vi "lead-lowPass_v8.vi"(7 "Enable?":bool, 9 "Denominator":fxp<+/-,18,3>[](array[numeric])=[0.0, 0.0], 10 "Numerator":fxp<+/-,18,3>[](array[numeric])=[0.0, 0.0], 11 "Input":fxp<+/-,25,4>) -> (3 "Output":fxp<+/-,25,4> format="%.29g")   [LabVIEW 2017, in "FPGA Controllers.lvlib"]
doc: "Lead controller with a low-pass filter, to have a -1 slope roll off.\n\nImplements, u(k) = a0*e(k-2) + a1*e(k-1) - b0*u(k-2) - b1*u(k-1)\n\nSet parameters, Num = a0, a1 and Den = b0, b1"
uses:
  FPGA Controllers.lvlib
  <vilib>/rvi/FXPMathLib/basic elements/FxpDiscreteDelay/XNode/nifxpmath_DiscreteDelay.xnode
  <vilib>/Platform/TimedLoop/XDataNode/XDataNode.xnode
  <vilib>/Platform/TimedLoop/XDataNode/nitl_modes.ctl
  <vilib>/Platform/TimedLoop/XDataNode/XDNodeRunTimeDep.lvlib
  <vilib>/Platform/TimedLoop/XDataNode/wakeup.ctl
  <vilib>/Platform/TimedLoop/XDataNode/timing_clust.ctl
  <vilib>/rvi/FXPMathLib/FxpMul/XNode/nifxpmath_Multiplier.xnode
  <vilib>/rvi/FXPMathLib/sim/FxpSim.dll
  <vilib>/rvi/FXPMathLib/FxpAdd/XNode/nifxpmath_Add.xnode
  <vilib>/rvi/FXPMathLib/FxpSub/XNode/nifxpmath_Sub.xnode
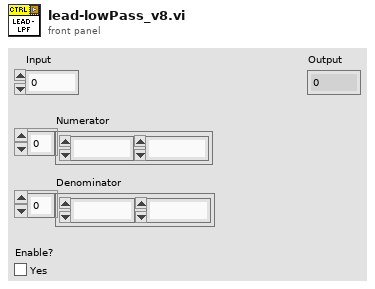
[diagram p1: front panel]
types:
  T1 = typedef "XDNodeRunTimeDep.lvlib/timing_clust.ctl" = cluster{"Expected End [f-1]":u64, "Actual End [f-1]":u64, "Finished Late? [f-1]":bool, "Expected End [i-1]":u64, "Actual End [i-1]":u64, "Finished Late? [i-1]":bool, "Expected Start [i]":u64, "Actual Start [i]":u64, "Expected Start [f]":u64, "Actual Start [f]":u64, "Source Name":string, "Structure Name":string, "Period":i64, "Deadline":i64, "Offset":i64, "Start":i64, "Priority":i32, "Timeout":i32, "Mode":T2, "Wakeup Reason":T3, "Error":errorcluster, "Source Type":string, "Secondary Source Type":string, "Global End Time":u64, "Global Start Time":u64, "Frame Duration":u64, "Iteration Duration":u64, "Assigned CPU":i32, "I/O Scan Engine Mode":u32}
  T2 = typedef "XDNodeRunTimeDep.lvlib/nitl_modes.ctl" = enum32{"No Change", "Process missed periods, maintain original phase", "Discard missed periods, maintain original phase", "Process missed periods, ignore original phase", "Discard missed periods, ignore original phase"}
  T3 = typedef "XDNodeRunTimeDep.lvlib/wakeup.ctl" = enum32{"Normal", "Aborted", "Asynchronous wakeup", "Timing source error", "Timed loop error", "Timeout"}
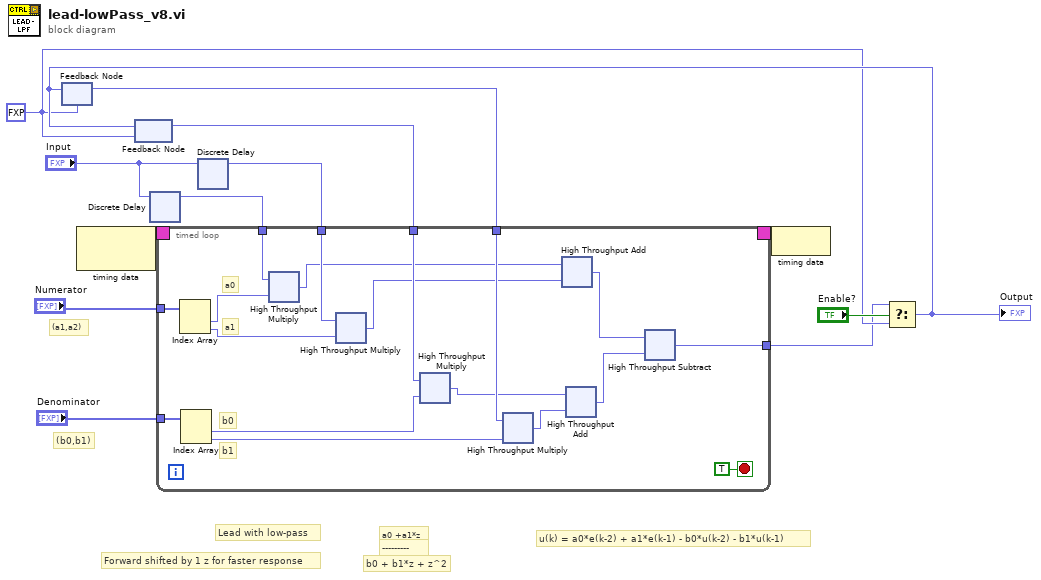
[diagram p0: block diagram]
diagram:
  w4 = fxp<+/-,25,4> 0.0 ("Input")
  # "u(k) = a0*e(k-2) + a1*e(k-1) - b0*u(k-2) - b1*u(k-1)"
  # "(b0,b1)"
  # "(a1,a2)"
  # "Forward shifted by 1 z for faster response"
  # "Lead with low-pass"
  # "b0 + b1*z + z^2"
  # "a0 +a1*z"
  # "---------"
  n1 = feedback #1(w4) -> (w5:fxp<+/-,25,4>)
  n2 = node-c288() -> (w11:T1)  [unwired: 1 in]
  n3 = feedback #2(w4) -> (w6:fxp<+/-,25,4>)
  n4 = xnode ("Discrete Delay")("D"="Input") -> ("Q"=w7:fxp<+/-,25,4>)
  n5 = xnode ("Discrete Delay")("D"="Input") -> ("Q"=w1:fxp<+/-,25,4>)
  n6 = timed-loop {
    timing: w11 -> [_]
    timing-out: [_] -> w10
    tunnel: "Numerator" -> [w30]
    tunnel: "Denominator" -> [w29]
    tunnel: w1 -> [w26]
    tunnel: w7 -> [w25]
    tunnel: w6 -> [w22]
    tunnel: w5 -> [w21]
    tunnel: [w14] -> w3
    stop <- TRUE stop-if-true
    # "b0"
    # "b1"
    # "a1"
    # "a0"
    n7 = Index Array(array=w30) -> (element #1=w28:fxp<+/-,18,3>, element #2=w27:fxp<+/-,18,3>)  [unwired: 2 in]
    n8 = Index Array(array=w29) -> (element #1=w23:fxp<+/-,18,3>, element #2=w24:fxp<+/-,18,3>)  [unwired: 2 in]
    n9 = xnode ("High Throughput Multiply")("x"=w25, "y"=w28) -> ("x*y"=w20:fxp<+/-,43,7>)
    n10 = xnode ("High Throughput Multiply")("x"=w26, "y"=w27) -> ("x*y"=w19:fxp<+/-,43,7>)
    n11 = xnode ("High Throughput Multiply")("x"=w22, "y"=w23) -> ("x*y"=w18:fxp<+/-,43,7>)
    n12 = xnode ("High Throughput Multiply")("x"=w21, "y"=w24) -> ("x*y"=w17:fxp<+/-,43,7>)
    n13 = xnode ("High Throughput Add")("x"=w20, "y"=w19) -> ("x+y"=w15:fxp<+/-,44,8>)
    n14 = xnode ("High Throughput Add")("x"=w18, "y"=w17) -> ("x+y"=w16:fxp<+/-,44,8>)
    n15 = xnode "High Throughput Subtract"("x"=w15, "y"=w16) -> ("x-y"=w14:fxp<+/-,25,4>)
  }
  n16 = node-c288(w10) -> ()
  n17 = Select(t=w3, s="Enable?", f=w4) -> (s? t:f=w12:fxp<+/-,25,4>)
  "Output" <- w12
  n18 = feedback-in #1(w12) -> ()
  n19 = feedback-in #2(w12) -> ()
